vi "AE_Set-file-properties.vi"(1 "Gain (dB)":dbl, 4 "error in (no error)":errorcluster, 5 "Rate (Hz)":dbl, 7 "text file":refnum<file>) -> (0 "error out":errorcluster, 3 "text file out":refnum<file>)   [LabVIEW 2012]
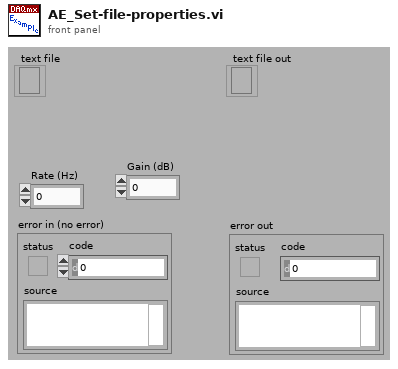
[diagram p1: front panel]
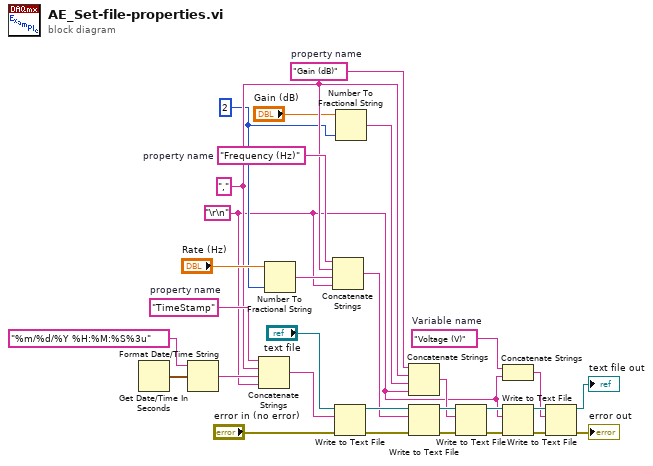
[diagram p0: block diagram]
diagram:
  w3 = "Voltage (V)"  # Variable name
  w10 = "Gain (dB)"  # property name
  w1 = "\r\n"
  w24 = "Frequency (Hz)"  # property name
  w6 = i16 2 ("precision (6)")
  w9 = "," ("delimiter (Tab)")
  w27 = "TimeStamp"  # property name
  n1 = Get Date/Time In Seconds() -> (seconds since 1Jan1904=w17:timestamp)
  n2 = Format Date/Time String(time format string (%c)="%m/%d/%Y %H:%M:%S%3u", seconds (now)=w17) -> (date/time string=w15:string)  [unwired: 1 in]
  n3 = Concatenate Strings(w27, w9, w15, w1) -> (w26:string)
  n4 = Number To Fractional String(number="Rate (Hz)", precision (6)=w6) -> (F-format string=w28:string)  [unwired: 2 in]
  n5 = Concatenate Strings(w24, w9, w28, w1) -> (w25:string)
  n6 = Write to Text File(file (use dialog)="text file", text=w26, error in="error in (no error)") -> (refnum out=w30:refnum<file>, error out=w29:errorcluster)  [unwired: 1 in, 1 out]
  n7 = Number To Fractional String(number="Gain (dB)", precision (6)=w6) -> (F-format string=w7:string)  [unwired: 2 in]
  n8 = Concatenate Strings(w10, w9, w7, w1) -> (w5:string)
  n9 = Write to Text File(file (use dialog)=w30, text=w25, error in=w29) -> (refnum out=w14:refnum<file>, error out=w13:errorcluster)  [unwired: 1 in, 1 out]
  n10 = Write to Text File(file (use dialog)=w14, text=w5, error in=w13) -> (refnum out=w11:refnum<file>, error out=w12:errorcluster)  [unwired: 1 in, 1 out]
  n11 = Concatenate Strings(w3, w1) -> (w2:string)
  n12 = Write to Text File(file (use dialog)=w11, text=w1, error in=w12) -> (refnum out=w23:refnum<file>, error out=w4:errorcluster)  [unwired: 1 in, 1 out]
  n13 = Write to Text File(file (use dialog)=w23, text=w2, error in=w4) -> (refnum out=→"text file out":refnum<file>, error out=→"error out":errorcluster)  [unwired: 1 in, 1 out]
